vi "PH_PowerUnit_BaseClass.PC InternalTiming.vi"(0 "i ref in":refnum<vi>, 2 "Waiting Time over? new":bool caption="Waiting Time over?", 3 "Waiting Time over? old":bool caption="Waiting Time over?", 5 "error in (no error)":errorcluster) -> (14 "i ref out":refnum<vi>, 19 "error out":errorcluster)   [LabVIEW 2014, in "PH_PowerUnit_BaseClass.lvlib"]
doc: "This VI writes the remaining time to the GUI object. If \"Required Device(s) off?\" is true, the GUI object blinks. The \"Waiting Over?\" is written to own attributes."
uses:
  PH_PowerUnit_BaseClass.lvlib
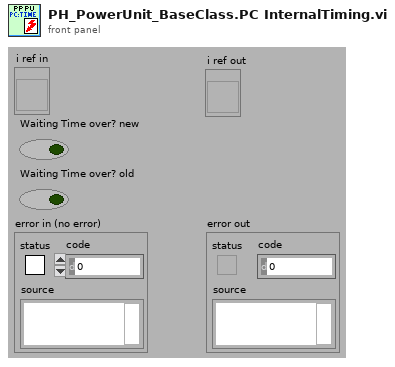
[diagram p1: front panel]
types:
  T1 = typedef "PH_PowerUnit_BaseClass.lvlib/PH_PowerUnit_BaseClass.i attribute.ctl" = cluster{"Constructor finished":bool, "PU":cluster{"In use":bool, "Service ID in use":i32, "GUI Ref":refnum<vi>}, "Enabling":cluster{"State":T2, "GUI Ref":refnum<vi>}, "Timing":cluster{"Last Shot":dbl, "Time between Shots [Sec]":dbl, "Waiting Time over?":bool, "Service ID Waiting Time":i32, "GUI Ref":refnum<vi>, "Instance":cluster{"Status":T3, "linked?":bool, "GUI Ref":refnum<vi>}}, "Sequencer":cluster{"SM State":string, "GUI Ref":refnum<vi>, "linked":bool}, "Subscribed Trendmssgs":cluster{"Tagname":string, "Status":T3, "linked?":bool, "Shot Condition":T3, "GUI Ref":refnum<vi>}[], "PP PU":T4, "Default Voltage (V)":dbl, "GUI Refs":T5, "PSDB data":cluster{"Shot Voltage [V]":dbl, "State TO SM":T6, "Write 2 early":bool}, "State TO SM":T6}
  T2 = typedef "PH_SystemInformation.lvlib/PH_SystemInformationEnabling State.ctl" = i32
  T3 = typedef "PH_StatusHandler.lvlib/PH_StatusHandler.Status.ctl" = i16
  T4 = typedef "PH_PP_Common.lvlib/PH_PP_Common.PUs.ctl" = enum16{"no Info", "PA-19mm-1", "PA-19mm-2", "PA-45mm-PILC", "PA-45mm-MAIN", "MA-PU-1", "MA-PU-2", "MA-PU-3", "MA-PU-4", "MA-PU-5", "MA-PU-6", "MA-FR", "MA-PILC", "PA-45mm-DP"}
  T5 = typedef "PH_PowerUnit_BaseClass.lvlib/PH_PowerUnit_BaseClass.GUI Refs.ctl" = cluster{"Delete Inst":refnum<vi>, "State TO SM":refnum<vi>, "State SM":refnum<vi>, "Fire":refnum<vi>}
  T6 = typedef "PH_PowerUnit_BaseClass.lvlib/PH_PowerUnit_BaseClass.SM States.ctl" = enum16{".", "Stand by", "Switch PU on", "Configure", "Set Default Voltage", "Set STANDBY", "Set READY", "Wait for Shot Cmd", "Open Dump Rods", "Open Ross Relais", "Close Ross Relais", "Switch PSU on", "Switch PSU off", "Charge", "Switch GD Channel on", "Close Dump Rods", "Rods-TO", "RR-TO", "PSU-TO", "Trigger-TO"}
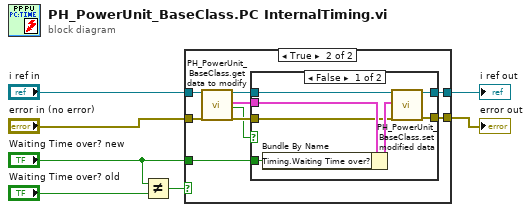
[diagram p0: block diagram]
diagram:
  n1 = Not Equal?(x="Waiting Time over? new", y="Waiting Time over? old") -> (x != y?=w3:bool)
  n2 = case shown="True" w3 {
    tunnel: "error in (no error)" -> [w8 w18]
    tunnel: "i ref in" -> [w9 w17]
    tunnel: [w9 w15] -> w5
    tunnel: [w8 w14] -> w4
    tunnel: "Waiting Time over? new" -> [_ w12]
    frame False {
    }
    frame True {
      n3 = call "PH_PowerUnit_BaseClass.get data to modify.vi"("i ref in"=w17, "error in (no error)"=w18) -> ("i ref out"=w16:refnum<vi>, "i attribute"=w13:T1, "timed out"=w10:bool, "error out"=w11:errorcluster)  [unwired: 14 in]
      n4 = case shown="False" w10 {
        tunnel: w16 -> [w25 w27]
        tunnel: [w24 w27] -> w15
        tunnel: [w23 w26] -> w14
        tunnel: w13 -> [w22 _]
        tunnel: w12 -> [w20 _]
        tunnel: w11 -> [w19 w26]
        frame False {
          n5 = Bundle By Name(cluster=w22, "Timing.Waiting Time over?"=w20) -> (w21:T1)
          n6 = call "PH_PowerUnit_BaseClass.set modified data.vi"("i ref in"=w25, "i attribute"=w21, "error in (no error)"=w19) -> ("i ref out"=w24:refnum<vi>, "error out"=w23:errorcluster)  [unwired: 15 in]
        }
        frame True {
        }
      }
    }
  }
  "error out" <- w4
  "i ref out" <- w5
